vi "SubConfocal_GetInfo.vi"(8 "Error In":errorcluster, 11 "Confocal line (VISA IN)":refnum<visa-resource-name>="COM1") -> (0 "Error out":errorcluster, 5 "Confocal Info":T1={"Actual Disk speed (rpm)"="3000", "Actual FW speed (rpm)"=3})   [LabVIEW 2015]
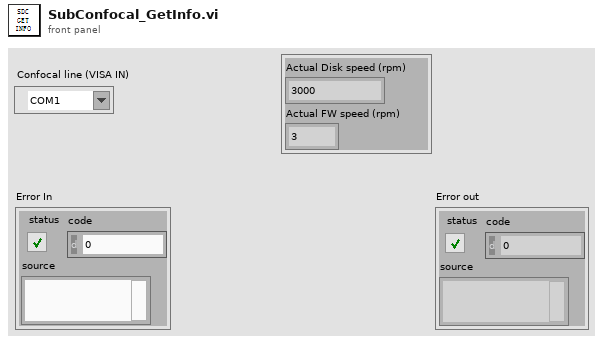
[diagram p1: front panel]
types:
  T1 = cluster{"Actual Disk speed (rpm)":string, "Actual FW speed (rpm)":i32}
  T2 = cluster{"Actual Disk speed (rpm)":string, "Actual FW speed":i32}
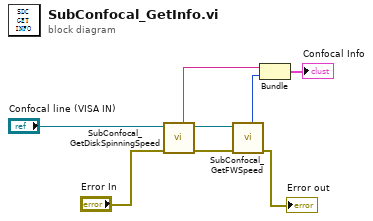
[diagram p0: block diagram]
diagram:
  n1 = call "SubConfocal_GetDiskSpinningSpeed.vi"("Error In"="Error In", "Confocal line (VISA IN)"="Confocal line (VISA IN)") -> ("Error out"=w6:errorcluster, "VISA OUT"=w7:refnum<visa-resource-name>, "Actual Disk speed (rpm)"=w5:string)  [unwired: 7 in]
  n2 = call "SubConfocal_GetFWSpeed.vi"("Error In"=w6, "Confocal line (VISA IN)"=w7) -> ("Error out"=→"Error out":errorcluster, "Actual FW speed"=w4:i32)  [unwired: 7 in, 1 out]
  n3 = Bundle("Actual Disk speed (rpm)"=w5, "Actual FW speed"=w4) -> (→"Confocal Info":T2)  [unwired: 1 in]
